vi "AIM664 Transmit Sampling Write.vi"() -> ()   [LabVIEW 2020]
uses:
  src/AIM664LV.lvlib
panel:
  in  "Data":u8[](array[numeric])=[5, 2, 5, 6, 4, 5, 6, 7, 8, 9]
  out "BytesWritten":u32
  out "TxStatus":T1 {"TransmitMode" items=["FDX_TX_GENERIC", "FDX_TX_REPLAY", "FDX_TX_INDIVIDUAL"]; "TxStatus" items=["FDX_STAT_STOP", "FDX_STAT_RUN", "FDX_STAT_ERROR", "FDX_STAT_WAIT_F_TRIG"]}
  in  "UdpDescription":T2={"PortType"=0, "UdpSrc"=0, "IpSrc"=167846145, "VlId"=0, "IpDst"=3772776448, "UdpDst"=1, "SubVlId"=1, "UdpNumBufMessages"=5, "UdpMaxMessageSize"=800, "UdpSamplingRate"=100} {"IpDst" format="%x"; "IpSrc" format="%x"}
  in  "TransmitMode":u32(ring)=2 items=["FDX_TX_GENERIC", "FDX_TX_REPLAY", "FDX_TX_INDIVIDUAL"]
  in  "Input":T3={"VlId"=0, "SubVls"=4, "Bag"=8, "NetSelect"=3, "MaxFrameLength"=1000, "FrameBufferSize"=0, "MACSourceLSLW"=35520, "MACSourceMSLW"=512, "Skew"=0} {"MACSourceMSLW" format="%x"; "NetSelect" items=["FDX_TX_FRAME_DLY_A"=0, "FDX_TX_FRAME_DLY_B"=1, "FDX_TX_FRAME_BOTH "=3, "FDX_TX_FRAME_ONLY_A"=4, "FDX_TX_FRAME_ONLY_B "=5]; "MACSourceLSLW" format="%x"}
  out "ResourceInfo":T4 {"PortMode" items=[" FDX_SINGLE", "FDX_REDUNDANT"]}
  in  "TxControl":T5 {"ExtendedStopMode" items=["FDX_ESTOP_NOT_USED", "FDX_ESTOP_EXT_TRG", "FDX_ESTOP_EXT_TRG_RESTART", "FDX_ESTOP_TIME"]; "StartMode" items=["FDX_STOP", "FDX_START", "FDX_START_TRG", "FDX_START_TIME"]}
  in  "Input":T5={"StartMode"=1, "Count"=0, "Sign"=0, "Day"=0, "Hour"=0, "Min"=0, "Second"=0, "MilliSec"=0, "MicroSec"=0, "ExtendedStopMode"=0, "TransmitTime"=0} {"ExtendedStopMode" items=["FDX_ESTOP_NOT_USED", "FDX_ESTOP_EXT_TRG", "FDX_ESTOP_EXT_TRG_RESTART", "FDX_ESTOP_TIME"]; "StartMode" items=["FDX_STOP", "FDX_START", "FDX_START_TRG", "FDX_START_TIME"]}
  in  "Input Cluster":T6={"SrvName"="local", "ResourceID"=1, "ResourceType"=0} {"ResourceType" items=["Board", "Port"]}
  out "Output Cluster 2":T7={"ResourceID"=1, "ResourceType"=0, "ResourceInfo"="AMC-FDX-B2", "StructId"=0}
  in  "ServerRElement":u32=1
  out "PortInitOut":T8={"PortConfig"=0, "PortUsed"=1, "GlobalMemFree"=62889696, "SharedMemFree"=16566232} {"PortConfig" items=["FDX_SINGLE", "FDX_REDUNDANT"]}
  in  "ClientInfo":T9={"SrvName"="local", "ClHostName"="local", "ClUser"="Roland", "ClApplication"="Test", "ClApplicationVersion"="V01.00", "ResourceID"=2, "Privileges"=4294967295} {"Privileges" items=["PRIVILEGES_ADMIN"=4294967295]}
  out "NuOfResources":u32=3
  in  "SrvName":string="local"
  out "NuOfServers":u32=1
  # "ARINC 664 Transmit Sampling Port (Write)"
  # "Overview: Configure the board to write into a Sampling Port.\nRequirement: At least one AIM ARINC-664 board with installed AIM ARINC 664 BSP.\nRestrictions: None.\nInstruction:\n1. Run the VI.\n2. Verify the results in the indicators."
  # "QueryServerResourceCvi"
  # "FdxInitCvi"
  # "CountServerResourcesCvi"
  # "GetServerResourcesCvi"
  # "FdxLoginCvi"
  # "FdxTxPortInitCvi"
  # "FdxTxModeControlCvi"
  # "FdxTxCreateVLCvi"
  # "FdxTxUDPCreatePortCvi"
  # "FdxTxUDPWritePortCvi"
  # "FdxTxControlCvi"
  # "FdxTxStatusCvi"
  # "FdxTxControlCvi"
  # "Input"
  # "Input"
  # "Output"
  # "TxControl"
  # "Output"
  # "Output"
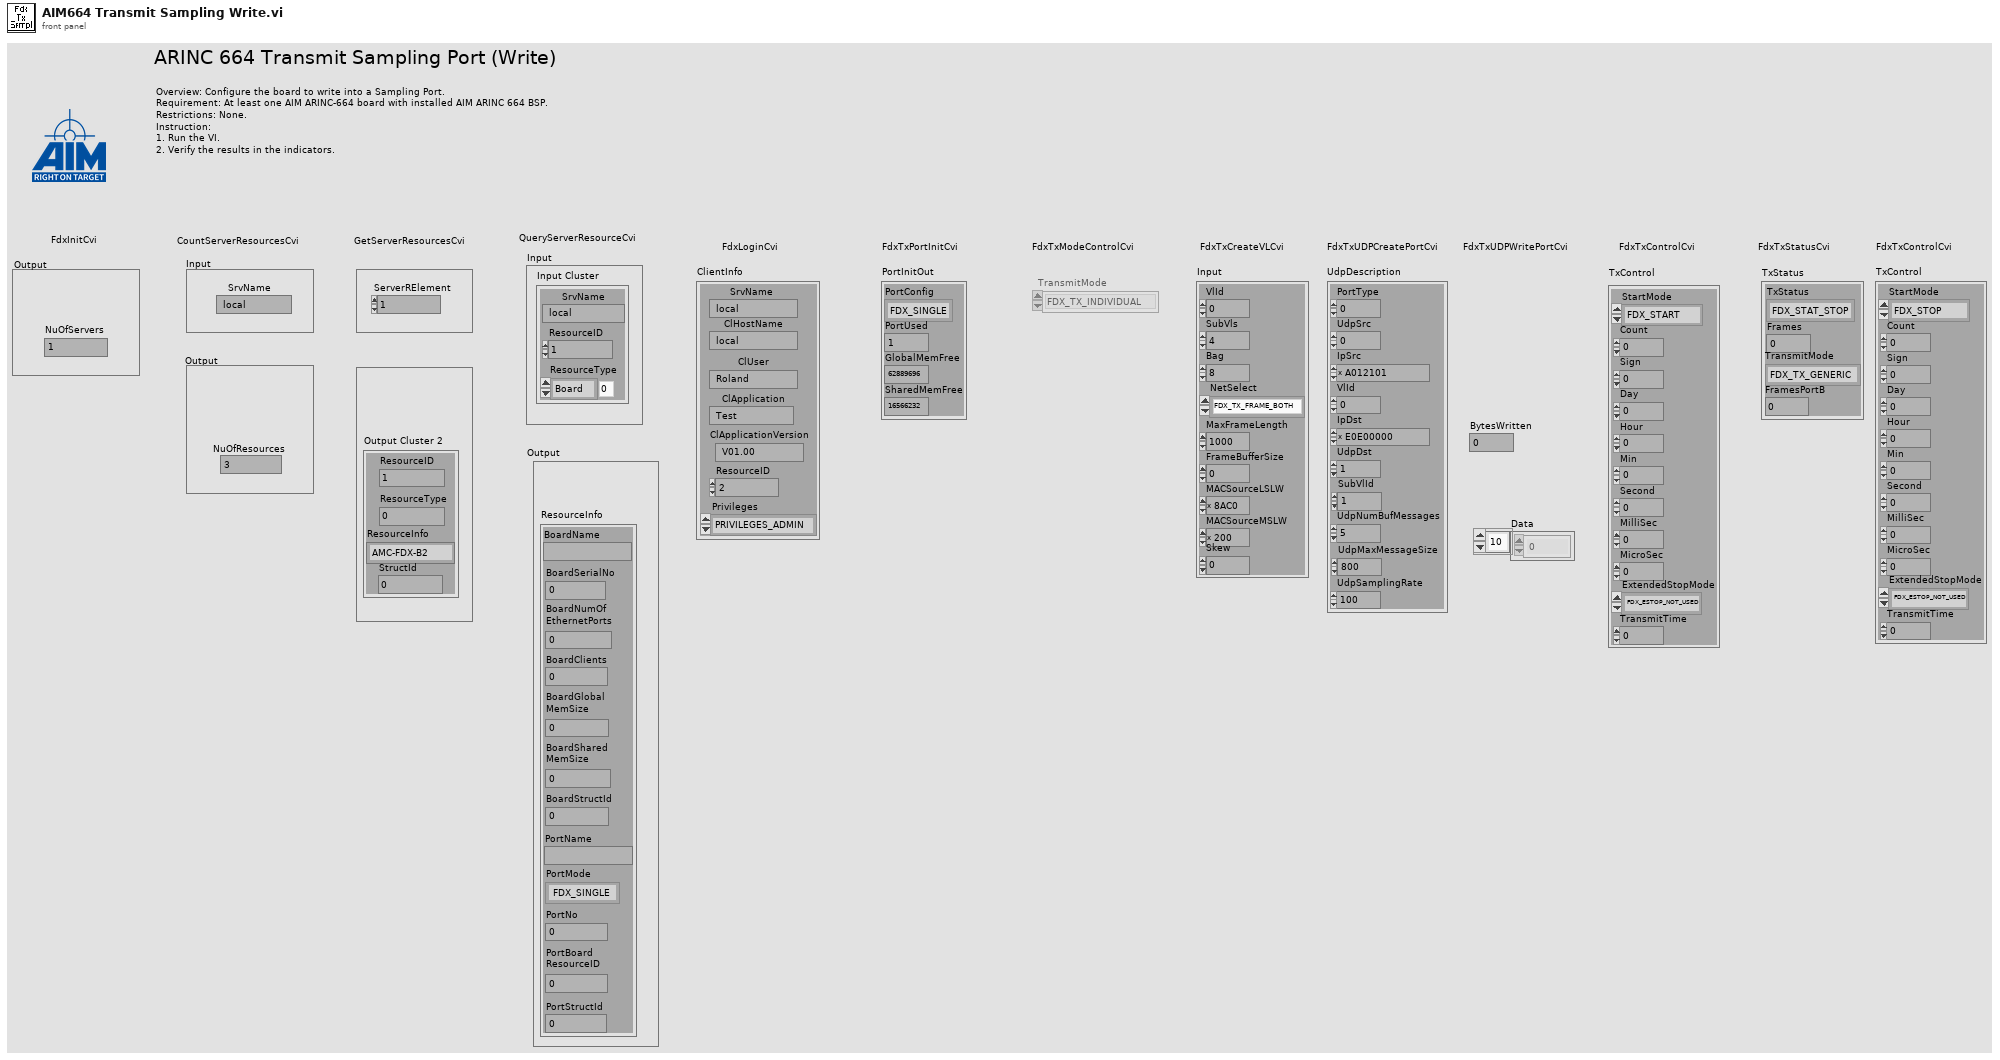
[diagram p1: front panel]
types:
  T1 = cluster{"TxStatus":u32, "Frames":u32, "TransmitMode":u32, "FramesPortB":u32}
  T2 = cluster{"PortType":u32, "UdpSrc":u32, "IpSrc":u32, "VlId":u32, "IpDst":u32, "UdpDst":u32, "SubVlId":u32, "UdpNumBufMessages":u32, "UdpMaxMessageSize":u32, "UdpSamplingRate":u32}
  T3 = cluster{"VlId":u32, "SubVls":u32, "Bag":u32, "NetSelect":u32, "MaxFrameLength":u32, "FrameBufferSize":u32, "MACSourceLSLW":u32, "MACSourceMSLW":u32, "Skew":u32}
  T4 = cluster{"BoardName":string, "BoardSerialNo":u32, "BoardNumOf\nEthernetPorts":u32, "BoardClients":u32, "BoardGlobal\nMemSize":u32, "BoardShared\nMemSize":u32, "BoardStructId":u32, "PortName":string, "PortMode":u32, "PortNo":u32, "PortBoard\nResourceID":u32, "PortStructId":u32}
  T5 = cluster{"StartMode":i32, "Count":u32, "Sign":i32, "Day":u32, "Hour":u32, "Min":u32, "Second":u32, "MilliSec":u32, "MicroSec":u32, "ExtendedStopMode":i32, "TransmitTime":u32}
  T6 = cluster{"SrvName":string, "ResourceID":u32, "ResourceType":u32}
  T7 = cluster{"ResourceID":u32, "ResourceType":u32, "ResourceInfo":string, "StructId":u32}
  T8 = cluster{"PortConfig":u32, "PortUsed":u32, "GlobalMemFree":u32, "SharedMemFree":u32}
  T9 = cluster{"SrvName":string, "ClHostName":string, "ClUser":string, "ClApplication":string, "ClApplicationVersion":string, "ResourceID":u32, "Privileges":u32}
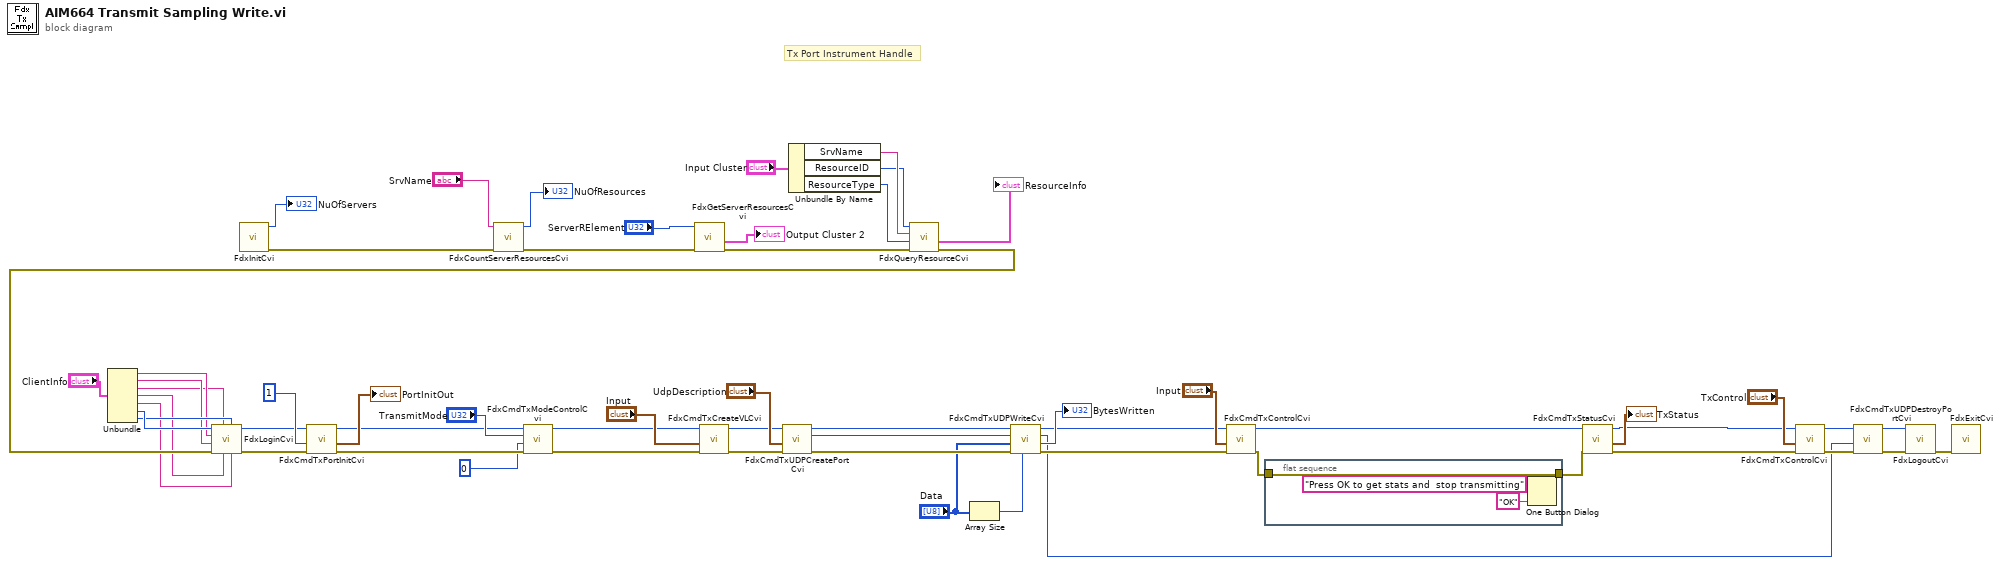
[diagram p0: block diagram]
diagram:
  # "Tx Port Instrument Handle"
  n1 = Unbundle("ClientInfo") -> ("SrvName"=w9:string, "ClHostName"=w8:string, "ClUser"=w7:string, "ClApplication"=w6:string, "ClApplicationVersion"=w5:string, "ResourceID"=w11:u32, "Privileges"=w10:u32)
  n2 = call "FdxInitCvi.vi"() -> ("error out"=w57:errorcluster, "Number of Servers"=→"NuOfServers":u32)  [unwired: 10 in]
  n3 = call "FdxCountServerResourcesCvi.vi"("error in"=w57, "SrvName (local)"="SrvName") -> ("error out"=w56:errorcluster, "Number of Resources"=→"NuOfResources":u32)  [unwired: 8 in]
  n4 = call "FdxGetServerResourcesCvi.vi"("error in"=w56, "ServerRElement"="ServerRElement") -> ("error out"=w51:errorcluster, "ServerResourceInfo"=→"Output Cluster 2":T7)  [unwired: 4 in, 4 out]
  n5 = Unbundle By Name("Input Cluster") -> ("SrvName"=w15:string, "ResourceID"=w14:u32, "ResourceType"=w13:u32)
  n6 = call "FdxQueryResourceCvi.vi"("error in"=w51, "ResourceType"=w13, "SrvName"=w15, "ResourceID"=w14) -> ("error out"=w50:errorcluster, "ResourceInfo"=→"ResourceInfo":T4)  [unwired: 5 in, 1 out]
  n7 = call "FdxLoginCvi.vi"("ClApplicationVersion"=w5, "Privileges"=w10, "ClApplication"=w6, "ClUser"=w7, "error in"=w50, "ClHostName"=w8, "SrvName"=w9, "ResourceID"=w11) -> ("error out"=w52:errorcluster, "InstrumentHandle"=w29:u32)  [unwired: 2 in]
  n8 = call "FdxCmdTxPortInitCvi.vi"("error in"=w52, "PortMap"=u32 1, "InstrumentHandle_port"=w29) -> ("error out"=w58:errorcluster, "PortInitOut"=→"PortInitOut":T8, "InstrumentHandle_port"=w28:u32)  [unwired: 6 in]
  n9 = call "FdxCmdTxModeControlCvi.vi"("error in"=w58, "RerosPortDelay"=u32 0, "TransmitMode"="TransmitMode", "InstrumentHandle_port"=w28) -> ("error out"=w54:errorcluster, "InstrumentHandle_port"=w27:u32)  [unwired: 6 in]
  n10 = call "FdxCmdTxCreateVLCvi.vi"("error in"=w54, "Input Cluster"="Input", "InstrumentHandle_port"=w27) -> ("error out"=w53:errorcluster, "InstrumentHandle_port"=w26:u32)  [unwired: 7 in]
  n11 = call "FdxCmdTxUDPCreatePortCvi.vi"("error in"=w53, "UdpDescription"="UdpDescription", "InstrumentHandle"=w26) -> ("error out"=w46:errorcluster, "UdpHandle"=w4:u32, "InstrumentHandle"=w25:u32)  [unwired: 6 in]
  n12 = Array Size(array="Data") -> (size(s)=w1:i32)
  n13 = call "FdxCmdTxUDPWriteCvi.vi"("ByteCount"=w1, "error in"=w46, "Data"="Data", "UdpHandle"=w4, "InstrumentHandle"=w25) -> ("error out"=w47:errorcluster, "BytesWritten"=→"BytesWritten":u32, "UdpHandle Out"=w3:u32, "InstrumentHandle"=w24:u32)  [unwired: 3 in]
  n14 = call "FdxCmdTxControlCvi.vi"("error in"=w47, "TxControl"="Input", "InstrumentHandle_port"=w24) -> ("error out"=w48:errorcluster, "InstrumentHandle_port"=w23:u32)  [unwired: 7 in]
  n15 = flat-sequence {
    tunnel: w48 -> [w61]
    tunnel: [w61] -> w45
    frame #0 {
      n16 = One Button Dialog(message="Press OK to get stats and  stop transmitting", button name ("OK")="OK") -> ()  [unwired: 1 out]
    }
  }
  n17 = call "FdxCmdTxStatusCvi.vi"("error in"=w45, "InstrumentHandle_port"=w23) -> ("error out"=w55:errorcluster, "TxStatus"=→"TxStatus":T1, "InstrumentHandle_port"=w22:u32)  [unwired: 7 in]
  n18 = call "FdxCmdTxControlCvi.vi"("error in"=w55, "TxControl"="TxControl", "InstrumentHandle_port"=w22) -> ("error out"=w44:errorcluster, "InstrumentHandle_port"=w21:u32)  [unwired: 7 in]
  n19 = call "FdxCmdTxUDPDestroyPortCvi.vi"("error in"=w44, "UdpHandle"=w3, "InstrumentHandle"=w21) -> ("error out"=w43:errorcluster, "InstrumentHandle"=w20:u32)  [unwired: 7 in]
  n20 = call "FdxLogoutCvi.vi"("error in"=w43, "InstrumentHandle"=w20) -> ("error out"=w49:errorcluster)  [unwired: 9 in]
  n21 = call "FdxExitCvi.vi"("error in"=w49) -> ()  [unwired: 10 in, 1 out]
